vi "Flightsimulator_S2_3.vi"() -> ()   [LabVIEW 2009]
uses:
  <vilib>/Platform/TimedLoop/XDataNode/XDataNode.xnode
  <vilib>/Platform/TimedLoop/XDataNode/loadlvalarms.vi
  <vilib>/Platform/TimedLoop/XDataNode/timing_clust.ctl
  <vilib>/Platform/TimedLoop/XDataNode/nitl_modes.ctl
  <vilib>/Platform/TimedLoop/XDataNode/wakeup.ctl
  <menus>/Universal Library/Das16.llb/FromEng(single).VI
  <vilib>/Platform/TimedLoop/XDataNode/XDNodeRunTimeDep.lvlib
  <vilib>/ptbypt/NI_PtbyPt.lvlib
panel:
  in  "Protocol123":u16(ring) items=["no color- no switch", "color mode", "no color- switch(black at change)"]
  out "colorchange":bool
  out "OK":bool=TRUE
  out "final test 2":dbl(slide)=-0.5605680868838764 scale=-1.0..1.0
  out "final test 1":dbl(slide)=0.24740124740124741 scale=-1.0..1.0
  out "training short":dbl(slide)=0.9652317880794702 scale=-1.0..1.0
  out "training8":dbl(slide)=0.9652317880794702 scale=-1.0..1.0
  out "training7":dbl(slide)=0.8611570247933884 scale=-1.0..1.0
  out "test3":dbl(slide)=-1.0 scale=-1.0..1.0
  out "training6":dbl(slide)=-0.21869782971619364 scale=-1.0..1.0
  out "training5":dbl(slide)=0.8540268456375839 max=5.904801692781309e-210 step=1.08742394e-315 scale=-1.0..1.0
  out "test 2":dbl(slide)=-0.6904962153069807 scale=-1.0..1.0
  out "test 1":dbl(slide)=-0.1886949293433084 scale=-1.0..1.0
  out "training 4":dbl(slide)=1.0 scale=-1.0..1.0
  out "training 3":dbl(slide)=1.0 scale=-1.0..1.0
  out "training 2":dbl(slide)=-0.2332214765100671 scale=-1.0..1.0
  out "training 1":dbl(slide)=0.03096234309623431 scale=-1.0..1.0
  out "pretest 2":dbl(slide)=-0.5708367854183927 scale=-1.0..1.0
  out "pretest 1":dbl(slide)=-0.26220016542597185 scale=-1.0..1.0
  out "protocol":string="nocolor mode"
  out "protocol 2":u16(ring)=1 items=["Switch mode", "color mode", "other"]
  in  "color":bool
  out "color when positive":string="green"
  in  "add to datainput":dbl
  in  "add period":dbl
  in  "forcelaseroffmanual":bool
  in  "minimumtotorquenotflying":ext
  in  "torquenotflying":ext=-6.216083831386964
  in  "beep":bool
  out "datatest":dbl=0.7859212239583333
  in  "DTC":bool=TRUE
  in  "minimum for not flying":ext=0.03
  in  "remarks":string="change in gain?"
  out "sleft01_right0-1":i32=-1
  out "period":i32=-12648 step=206880616
  out "ErrCode 3":i32
  out "laser power real":dbl=2.1
  in  "laser power 0-41":dbl=29.0
  in  "force laser on":bool
  out "laserison":bool
  out "laser":bool
  out "ErrCode 2":i32
  out "ErrCode":i32
  out "PULSE":bool
  out "error out 3":errorcluster
  in  "force end of exp":bool
  out "Elapsed Time (s) 2":dbl(slide)=43.1674690246582 caption="Elapsed Time (s)" max=1.19698869e-315 scale=0.12..120.0
  out "Score 2":dbl=0.17155756207674944
  out "Histogram 2":dynamicdata(graph)=[{"t0"=timestamp(-4.833333333333333 s since 1904-01-01), "dt"=0.3333333333333333, "Y"=[0.0, 0.0, 1.0, 3.0, 5.0, 9.0, 19.0, 14.0, 25.0, 26.0, 42.0, 53.0, 52.0, 68.0, 50.0, 11.0, 12.0, 28.0, 15.0, 30.0, 27.0, 39.0, 57.0, 65.0, 78.0, 157.0, 0.0, 0.0, 0.0, 0.0], "attributes"=variant("NI_ChannelName"=variant(string " (Histogram)"), "NI_ExpIsRelativeTime"=variant(bool TRUE), "NI_ExpStartTimeStamp"=variant(timestamp timestamp(0 s since 1904-01-01)), "NI_ExpTimeStamp"=variant(timestamp timestamp(3352812616.4418974 s since 1904-01-01)), "NI_ExpXDimension"=variant(string "BIN"), "NI_OriginalChannelName"=variant(string ""))}] caption="Histogram"
  out "Waveform Chart 3":ext(graph)=0.7863281249999999889
  out "end of experiment":bool
  out "punished":string="positive-left"
  out "Eng Units":sgl=0.78632814
  in  "serie(s)":dbl=60.0
  in  "genotype":string="wtb"
  in  "Path":path=path "D:/dokumente/data/FSdata/switcheffect/switch.txt"
  in  "side punished":bool=TRUE
  in  "start":bool
  # "left"
  # "right"
  # "x"
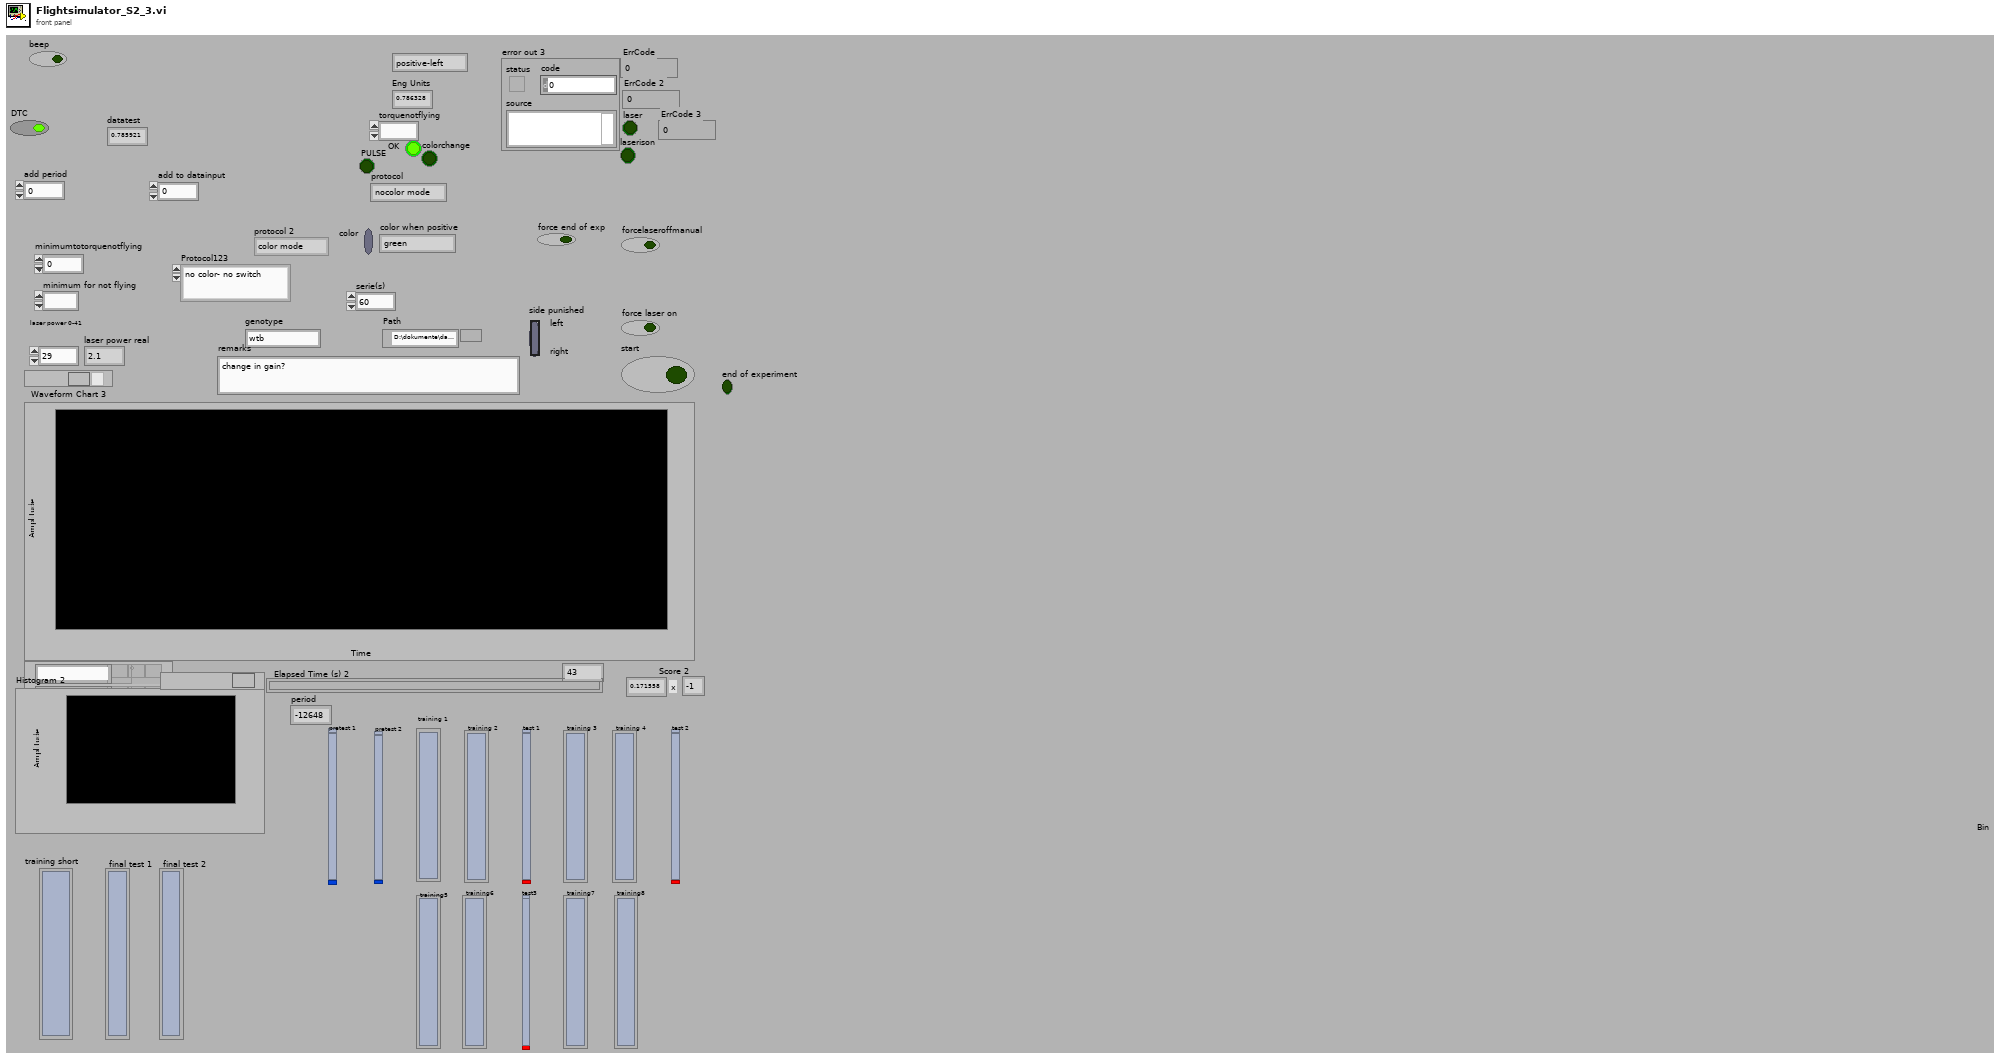
[diagram p1: front panel]
types:
  T1 = typedef "XDNodeRunTimeDep.lvlib/timing_clust.ctl" = cluster{"Expected End [f-1]":u64, "Actual End [f-1]":u64, "Finished Late? [f-1]":bool, "Expected End [i-1]":u64, "Actual End [i-1]":u64, "Finished Late? [i-1]":bool, "Expected Start [i]":u64, "Actual Start [i]":u64, "Expected Start [f]":u64, "Actual Start [f]":u64, "Source Name":string, "Structure Name":string, "Period":i64, "Deadline":i64, "Offset":i64, "Start":i64, "Priority":i32, "Timeout":i32, "Mode":T2, "Wakeup Reason":T3, "Error":errorcluster, "Source Type":string, "Secondary Source Type":string, "Global End Time":u64, "Global Start Time":u64, "Frame Duration":u64, "Iteration Duration":u64, "Assigned CPU":i32, "I/O Scan Engine Mode":u32}
  T2 = typedef "XDNodeRunTimeDep.lvlib/nitl_modes.ctl" = enum32{"No Change", "Process missed periods, maintain original phase", "Discard missed periods, maintain original phase", "Process missed periods, ignore original phase", "Discard missed periods, ignore original phase"}
  T3 = typedef "XDNodeRunTimeDep.lvlib/wakeup.ctl" = enum32{"Normal", "Aborted", "Asynchronous wakeup", "Timing source error", "Timed loop error", "Timeout"}
  T4 = enum16{"open", "replace", "create", "open or create", "replace or create", "replace or create with confirmation"}
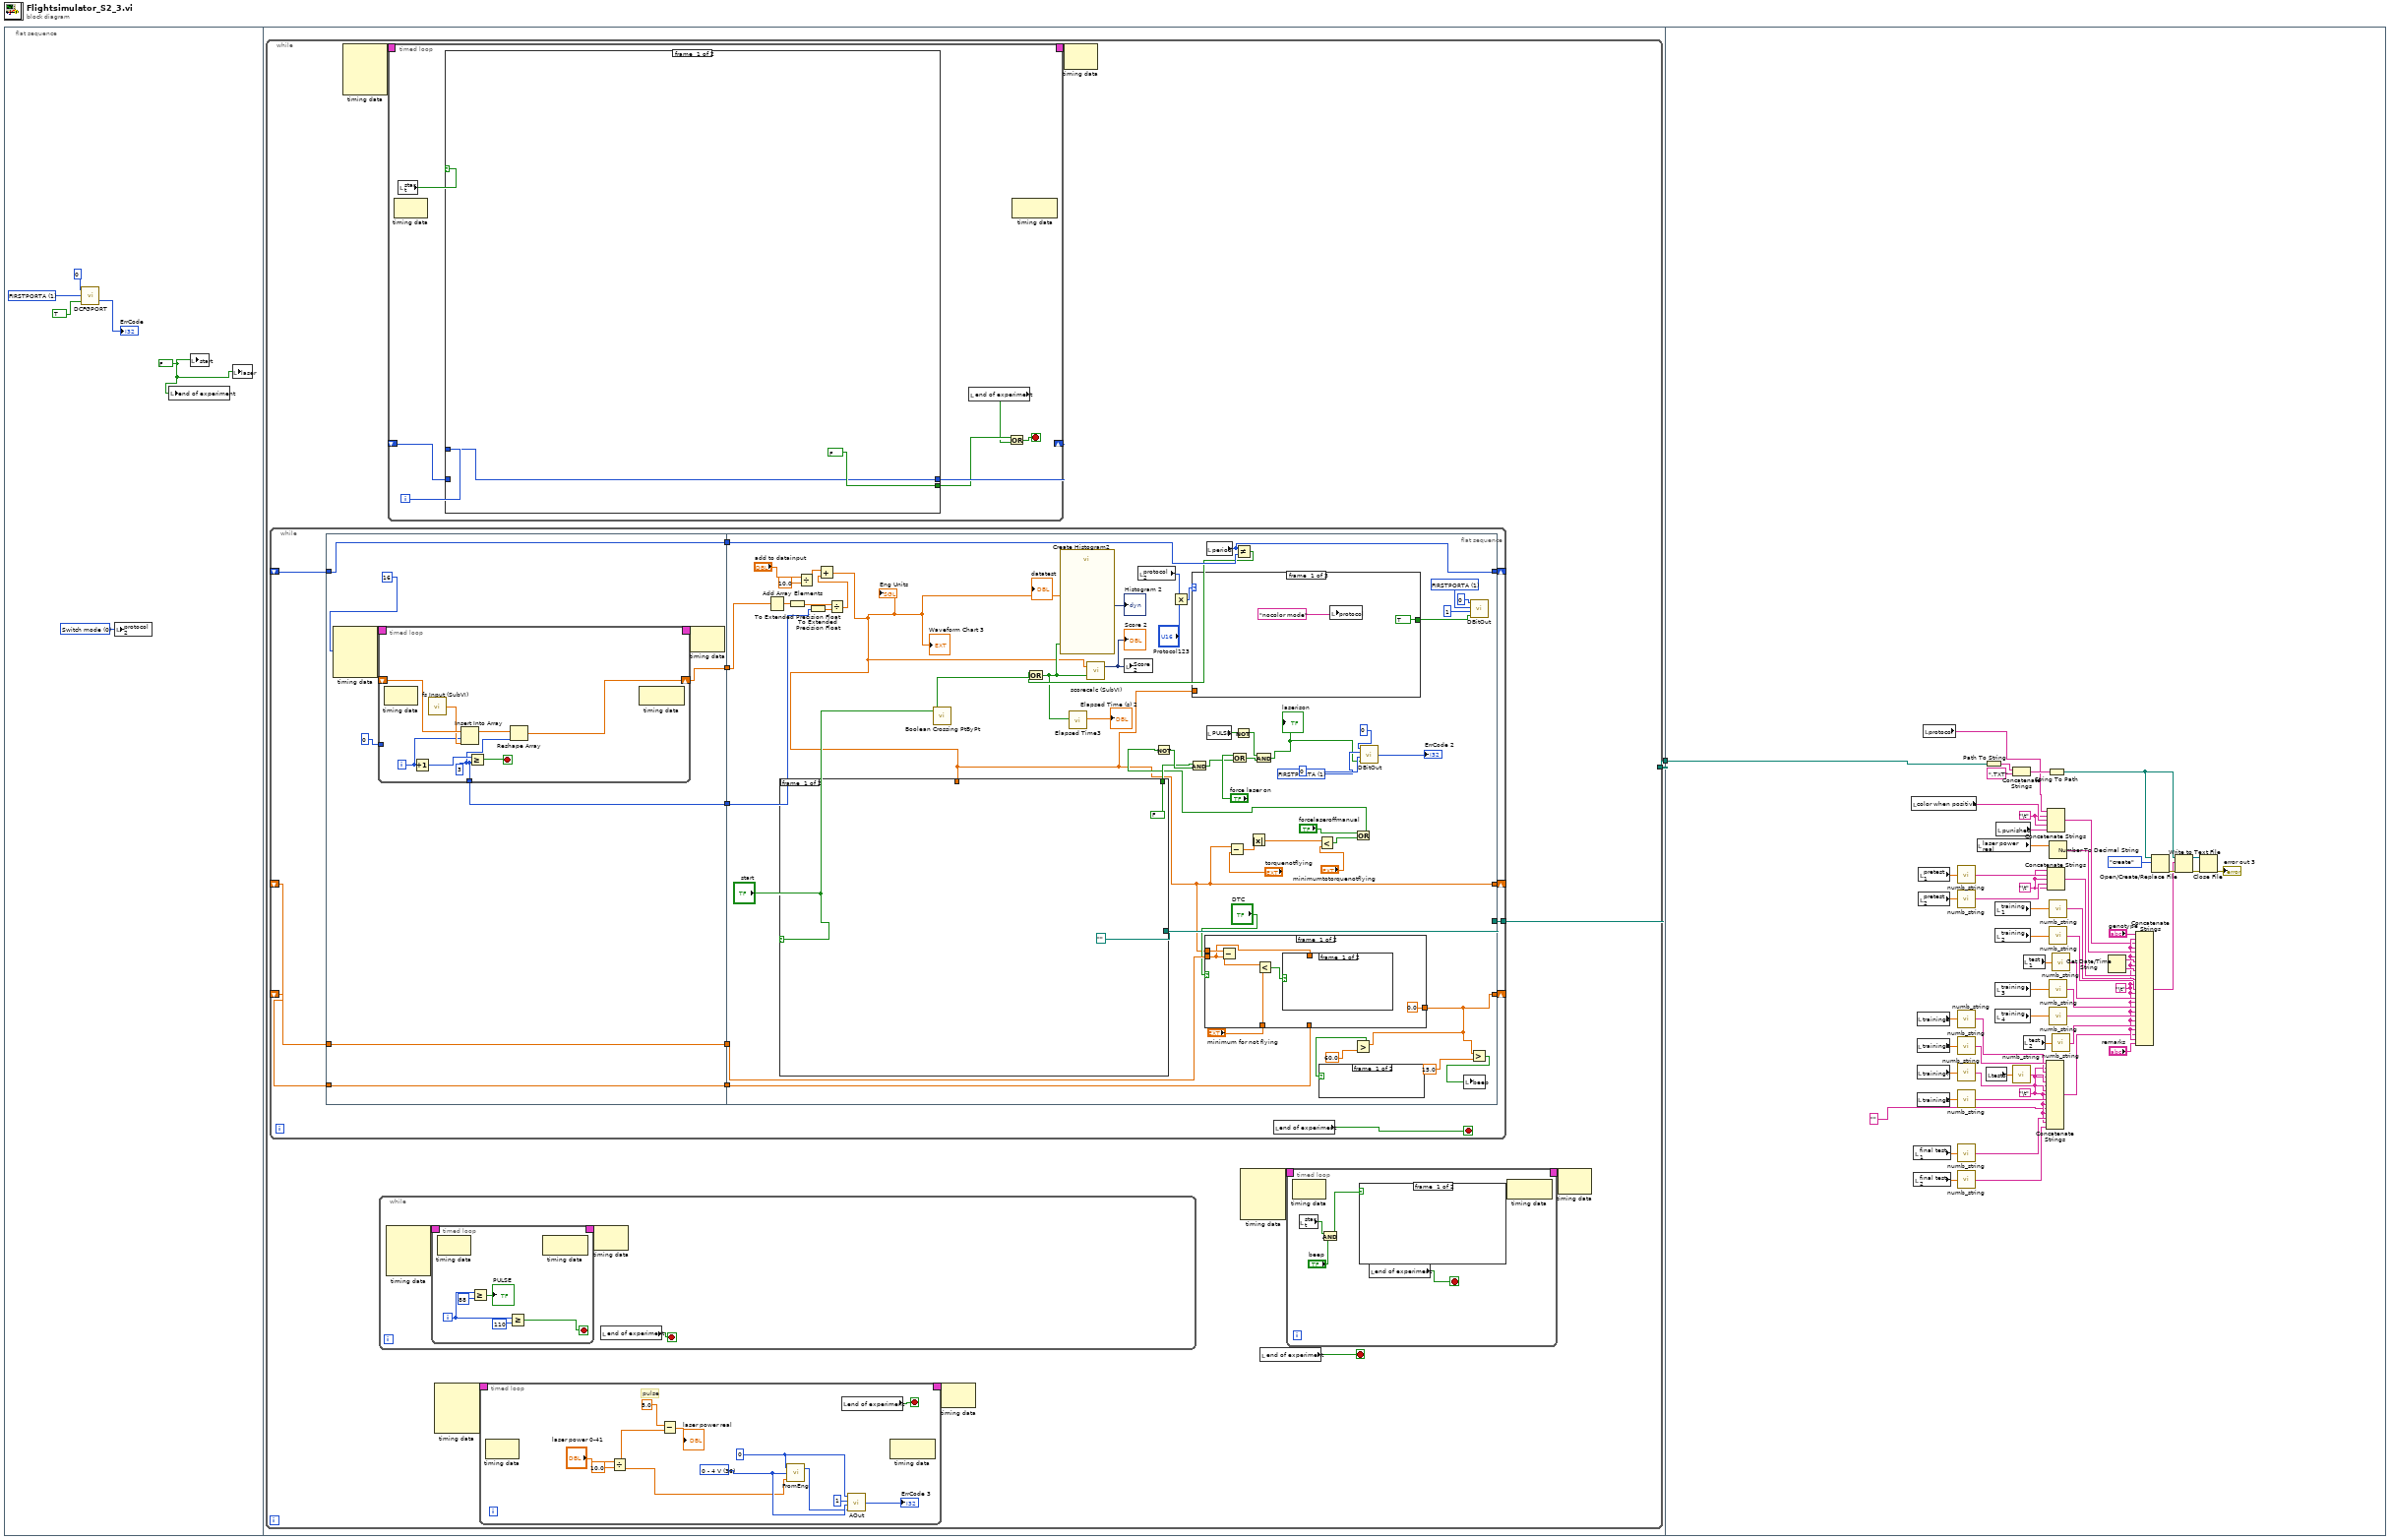
[diagram p0: block diagram]
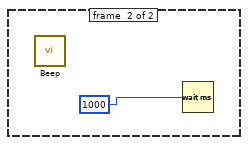
[diagram p2: hidden frame]
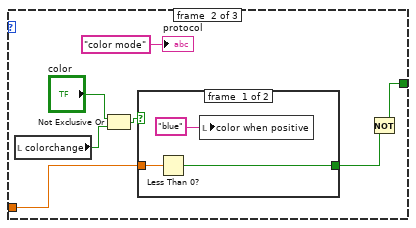
[diagram p3: hidden frame]
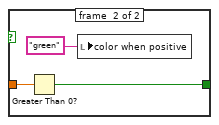
[diagram p4: hidden frame]
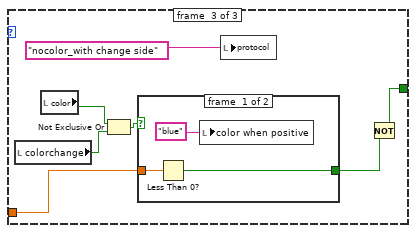
[diagram p5: hidden frame]
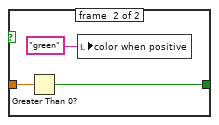
[diagram p6: hidden frame]
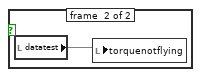
[diagram p7: hidden frame]
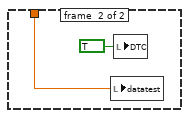
[diagram p8: hidden frame]
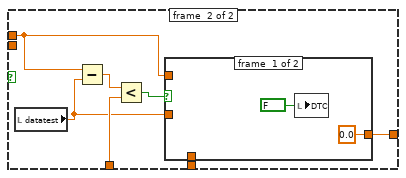
[diagram p9: hidden frame]
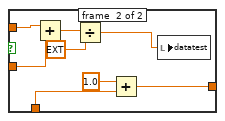
[diagram p10: hidden frame]
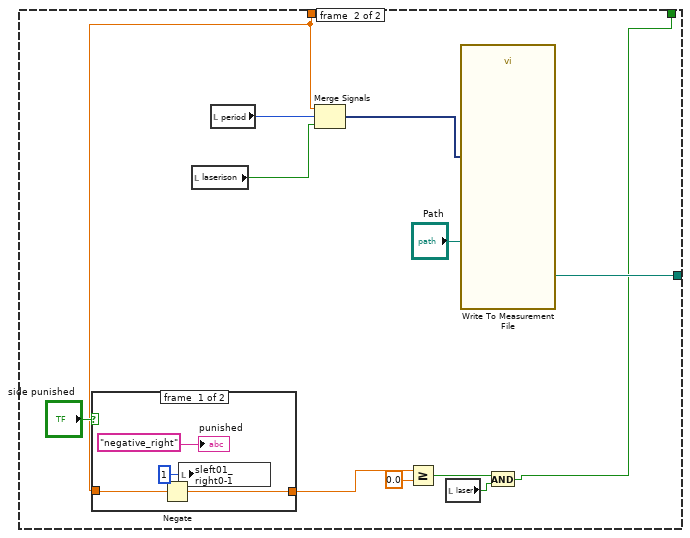
[diagram p11: hidden frame]
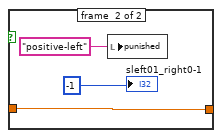
[diagram p12: hidden frame]
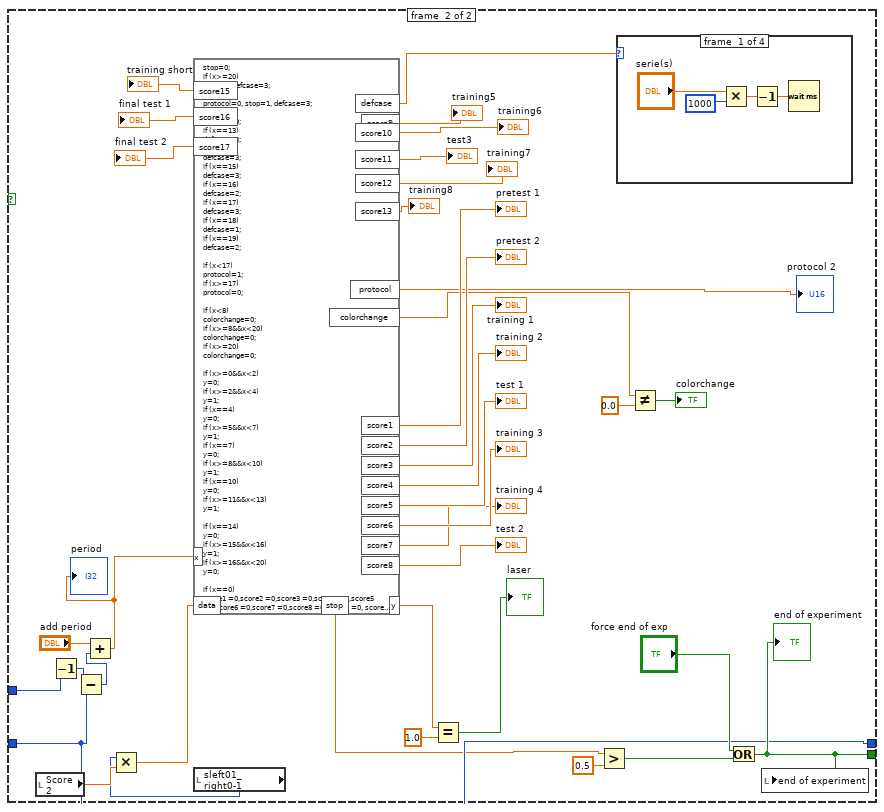
[diagram p13: hidden frame]
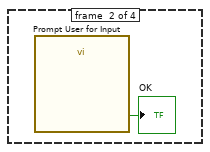
[diagram p14: hidden frame]
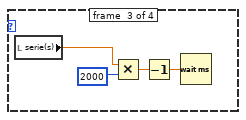
[diagram p15: hidden frame]
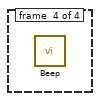
[diagram p16: hidden frame]
diagram:
  n1 = flat-sequence {
    tunnel: [w8] -> w1
    tunnel: w1 -> [w316]
    frame #0 {
      w2 = u16 0 items=["Switch mode", "color mode", "other"] ("protocol 2")
      w6 = 1 items=["AUXPORT", "FIRSTPORTA", "FIRSTPORTB", "FIRSTPORTCL", "FIRSTPORTCH", "SECONDPORTA", "SECONDPORTB", "SECONDPORTCL", "SECONDPORTCH", "THIRDPORTA", "THIRDPORTB", "THIRDPORTCL", "THIRDPORTCH", "FOURTHPORTA", "FOURTHPORTB", "FOURTHPORTCL", "FOURTHPORTCH", "FIFTHPORTA", "FIFTHPORTB", "FIFTHPORTCL", "FIFTHPORTCH", "SIXTHPORTA", "SIXTHPORTB", "SIXTHPORTCL", "SIXTHPORTCH", "SEVENTHPORTA", "SEVENTHPORTB", "SEVENTHPORTCL", "SEVENTHPORTCH", "EIGTHPORTA", "EIGHTHPORTB", "EIGHTHPORTCL", "EIGHTHPORTCH"] ("PortNum")
      w3 = FALSE
      n2 = call <menus>:"DCFGPORT.VI"("Direction"=TRUE, "PortNum"=w6, "BoardNum"=u32 0) -> ("ErrCode"=→"ErrCode":i32)  [unwired: 1 out]
      n3 = local write "protocol 2"(w2) -> ()
      n4 = local write "end of experiment"(w3) -> ()
      n5 = local write "start"(w3) -> ()
      n6 = local write "laser"(w3) -> ()
    }
    frame #1 {
      n7 = while {
        tunnel: [w11] -> w8
        stop <- w14 stop-if-true
        n8 = while {
          tunnel: [w53] -> w11
          shift-right: [w51] -> _
          shift-left: _ -> [w50]
          shift-right: [w46] -> _
          shift-left: _ -> [w44]
          shift-right: [w43] -> _
          shift-left: _ -> [w41]
          stop <- w52 stop-if-true
          n9 = flat-sequence {
            tunnel: [w60] -> w49
            tunnel: [w59] -> w48
            tunnel: [w56] -> w47
            tunnel: w50 -> [w56]
            tunnel: [w55] -> w45
            tunnel: w44 -> [w55]
            tunnel: [w54] -> w42
            tunnel: w41 -> [w54]
            tunnel: [w131] -> w53
            tunnel: w49 -> [w124]
            tunnel: w48 -> [w123]
            tunnel: [w116] -> w51
            tunnel: w47 -> [w115]
            tunnel: [w87] -> w46
            tunnel: w45 -> [w107]
            tunnel: [w98] -> w43
            tunnel: w42 -> [w105]
            frame #0 {
              n10 = node-c288(i64 16 ("Period")) -> (w62:T1)  [unwired: 3 in]
              n11 = timed-loop {
                tunnel: 0 ("y") -> [_]
                shift-right: [w66] -> w60
                shift-left: _ -> [w69]
                timing: w62 -> [_]
                timing-out: [_] -> w61
                tunnel: [w63] -> w59
                i -> [w64]
                stop <- w70 stop-if-true
                w63 = 3 ("y")
                n12 = node-c288() -> ()  [unwired: 1 in, 1 out]
                n13 = Increment(x=w64) -> (x+1=w65:i32)
                n14 = call "fs Input (SubVI).vi"() -> ("Eng Units"=w68:sgl)  [unwired: 1 out]
                n15 = Insert Into Array(array=w69, index=w64, new element=w68) -> (w67:sgl[])
                n16 = Greater Or Equal?(x=w65, y=w63) -> (x >= y?=w70:bool)
                n17 = Reshape Array(w67, w63) -> (w66:sgl[])
                n18 = node-c288() -> ()  [unwired: 1 in, 1 out]
              }
              n19 = node-c288(w61) -> ()  [unwired: 1 out]
            }
            frame #1 {
              w84 = u32 1 items=["AUXPORT", "FIRSTPORTA"] ("PortType")
              w120 = u32 1 items=["AUXPORT", "FIRSTPORTA"] ("PortType")
              n20 = Add Array Elements(numeric array=w124) -> (sum=w127:sgl)
              n21 = To Extended Precision Float(1:w127) -> (0:w125:ext)
              n22 = Divide(x="add to datainput", y=10.0) -> (x/y=w79:dbl)
              n23 = To Extended Precision Float(1:w123) -> (0:w126:ext)
              n24 = Divide(x=w125, y=w126) -> (x/y=w88:ext)
              n25 = Add(x=w79, y=w88) -> (x+y=w87:ext)
              "Eng Units" <- w87
              "Waveform Chart 3" <- w87
              n26 = case shown="True" "start" {
                tunnel: w87 -> [_ w191]
                tunnel: [path "" ("Filename Out") w197] -> w131
                tunnel: [FALSE w188] -> w100
                frame #0 {
                }
                frame #1 {
                  n27 = case shown="False" "side punished" {
                    tunnel: w191 -> [w203 w206]
                    tunnel: [w201 w206] -> w196
                    frame #0 {
                      n28 = Negate(x=w203) -> (-x=w201:ext)
                      n29 = local write "sleft01_right0-1"(1 ("sleft01_right0-1")) -> ()
                      "punished" <- "negative_right"
                    }
                    frame #1 {
                      n30 = local write "punished"("positive-left") -> ()
                      "sleft01_right0-1" <- -1
                    }
                  }
                  n31 = local read "laserison"() -> (w189:bool)
                  n32 = local read "period"() -> (w190:i32)
                  n33 = Merge Signals(w191, w190, w189) -> (w198:dynamicdata)
                  n34 = Greater Or Equal?(x=w196, y=sgl 0.0) -> (x >= y?=w193:bool)
                  n35 = local read "laser"() -> (w192:bool)
                  n36 = call "Write To Measurement File"("Signals"=w198, "Filename"="Path") -> ("Filename Out"=w197:path)  [unwired: 15 in, 2 out]
                  n37 = And(x=w193, y=w192) -> (x .and. y?=w188:bool)
                }
              }
              n38 = call <vilib>:"Boolean Crossing PtByPt.vi"("input"="start") -> ("crossing"=w129:bool)  [unwired: 2 in]
              n39 = local read "protocol 2"() -> (w82:u16)
              n40 = Multiply(x="Protocol123", y=w82) -> (x*y=w81:u16)
              n41 = case shown="2" w81 {
                tunnel: w87 -> [_ w138 w152]
                tunnel: [TRUE w136 w151] -> w83
                frame #0 {
                  n42 = local write "protocol"("nocolor mode") -> ()
                }
                frame #1 {
                  n43 = local read "colorchange"() -> (w134:bool)
                  n44 = Not Exclusive Or(1:w134, 2:"color") -> (0:w135:bool)
                  n45 = case shown="True" w135 {
                    tunnel: [w143 w146] -> w140
                    tunnel: w138 -> [w141 w144]
                    frame #0 {
                      n46 = Less Than 0?(x=w141) -> (x < 0?=w143:bool)
                      n47 = local write "color when positive"("blue") -> ()
                    }
                    frame #1 {
                      n48 = Greater Than 0?(x=w144) -> (x > 0?=w146:bool)
                      n49 = local write "color when positive"("green") -> ()
                    }
                  }
                  n50 = Not(x=w140) -> (.not. x?=w136:bool)
                  "protocol" <- "color mode"
                }
                frame #2 {
                  n51 = local read "colorchange"() -> (w149:bool)
                  n52 = local read "color"() -> (w148:bool)
                  n53 = Not Exclusive Or(1:w149, 2:w148) -> (0:w150:bool)
                  n54 = case shown="True" w150 {
                    tunnel: [w156 w159] -> w153
                    tunnel: w152 -> [w154 w157]
                    frame #0 {
                      n55 = Less Than 0?(x=w154) -> (x < 0?=w156:bool)
                      n56 = local write "color when positive"("blue") -> ()
                    }
                    frame #1 {
                      n57 = Greater Than 0?(x=w157) -> (x > 0?=w159:bool)
                      n58 = local write "color when positive"("green") -> ()
                    }
                  }
                  n59 = local write "protocol"("nocolor_with change side") -> ()
                  n60 = Not(x=w153) -> (.not. x?=w151:bool)
                }
              }
              n61 = case shown="True" "DTC" {
                tunnel: "minimum for not flying" -> [w165 w174]
                tunnel: w107 -> [w161 _]
                tunnel: w87 -> [w164 w169]
                tunnel: w105 -> [_ w171]
                tunnel: [0.0 w170] -> w98
                frame #0 {
                  n62 = Subtract(x=w164, y=w161) -> (x-y=w166:ext)
                  n63 = Less?(x=w166, y=w165) -> (x < y?=w163:bool)
                  n64 = case shown="True" w163 {
                    tunnel: w161 -> [_ w167]
                    frame #0 {
                    }
                    frame #1 {
                      n65 = local write "datatest"(w167) -> ()
                      n66 = local write "DTC"(TRUE ("DTC")) -> ()
                    }
                  }
                }
                frame #1 {
                  n67 = local read "datatest"() -> (w172:dbl)
                  n68 = Subtract(x=w169, y=w172) -> (x-y=w175:ext)
                  n69 = Less?(x=w175, y=w174) -> (x < y?=w173:bool)
                  n70 = case shown="True" w173 {
                    tunnel: w172 -> [_ w185]
                    tunnel: w169 -> [_ w184]
                    tunnel: w171 -> [_ w180]
                    tunnel: [0.0 w178] -> w170
                    frame #0 {
                      n71 = local write "DTC"(FALSE ("DTC")) -> ()
                    }
                    frame #1 {
                      n72 = Add(x=w184, y=w185) -> (x+y=w183:ext)
                      n73 = Divide(x=w183, y=ext 2.0) -> (x/y=w181:ext)
                      n74 = Add(x=1.0, y=w180) -> (x+y=w178:dbl)
                      n75 = local write "datatest"(w181) -> ()
                    }
                  }
                }
              }
              n76 = local read "period"() -> (w116:i32)
              n77 = local read "PULSE"() -> (w114:bool)
              n78 = Subtract(x=w87, y="torquenotflying") -> (x-y=w94:ext)
              n79 = Not(x=w114) -> (.not. x?=w113:bool)
              n80 = Not Equal?(x=w116, y=w115) -> (x != y?=w110:bool)
              n81 = Or(x=w110, y=w129) -> (x .or. y?=w103:bool)
              n82 = call "Create Histogram2"("Reset"=w103, "Signal"=w87) -> ("Histogram"=→"Histogram 2":dynamicdata)  [unwired: 8 in, 1 out]
              n83 = call "Elapsed Time3"("Reset"=w103) -> ("Elapsed Time (s)"=→"Elapsed Time (s) 2":dbl)  [unwired: 11 in, 7 out]
              n84 = call "scorecalc (SubVI).vi"("Reset"=w103, "Slide"=w87) -> ("Dynamic Data"=w128:dynamicdata)  [unwired: 1 out]
              "Score 2" <- w128
              n85 = local write "Score 2"(w128) -> ()
              n86 = Absolute Value(x=w94) -> (abs(x)=w89:ext)
              n87 = Less?(x=w89, y="minimumtotorquenotflying") -> (x < y?=w92:bool)
              n88 = Or(x="forcelaseroffmanual", y=w92) -> (x .or. y?=w90:bool)
              n89 = Not(x=w90) -> (.not. x?=w109:bool)
              n90 = And(x=w100, y=w109) -> (x .and. y?=w99:bool)
              n91 = Or(x="force laser on", y=w99) -> (x .or. y?=w112:bool)
              n92 = And(x=w113, y=w112) -> (x .and. y?=w101:bool)
              "laserison" <- w101
              n93 = Greater?(x=w98, y=60.0) -> (0:w96:bool)
              n94 = case shown="True" w96 {
                frame #0 {
                }
                frame #1 {
                  n95 = local read "datatest"() -> (w160:dbl)
                  n96 = local write "torquenotflying"(w160) -> ()
                }
              }
              n97 = call <menus>:"DBitOut.VI"("BitValue"=w101, "BitNum"=u32 0, "PortType"=w120, "BoardNum"=u32 0) -> ("ErrCode"=→"ErrCode 2":i32)
              n98 = Greater?(x=w98, y=15.0) -> (0:w102:bool)
              n99 = local write "beep"(w102) -> ()
              n100 = call <menus>:"DBitOut.VI"("BitValue"=w83, "BitNum"=u32 1, "PortType"=w84, "BoardNum"=u32 0) -> ()  [unwired: 1 out]
            }
          }
          n101 = local read "end of experiment"() -> (w52:bool)
        }
        n102 = node-c288() -> (w16:T1)  [unwired: 4 in]
        n103 = while {
          stop <- w207 stop-if-true
          n104 = node-c288() -> (w209:T1)  [unwired: 4 in]
          n105 = timed-loop {
            timing: w209 -> [_]
            timing-out: [_] -> w208
            i -> [w212]
            stop <- w210 stop-if-true
            n106 = node-c288() -> ()  [unwired: 1 in, 1 out]
            n107 = Greater Or Equal?(x=w212, y=88 ("SIZE1")) -> (x >= y?=→"PULSE":bool)
            n108 = Greater Or Equal?(x=w212, y=110 ("RESET PULSE")) -> (x >= y?=w210:bool)
            n109 = node-c288() -> ()  [unwired: 1 in, 1 out]
          }
          n110 = node-c288(w208) -> ()  [unwired: 1 out]
          n111 = local read "end of experiment"() -> (w207:bool)
        }
        n112 = timed-loop {
          timing: w16 -> [_]
          timing-out: [_] -> w15
          shift-right: [w222] -> _
          shift-left: _ -> [w223]
          i -> [w224]
          stop <- w220 stop-if-true
          n113 = node-c288() -> ()  [unwired: 1 in, 1 out]
          n114 = local read "start"() -> (w225:bool)
          n115 = case shown="True" w225 {
            tunnel: [FALSE w263] -> w221
            tunnel: w224 -> [w226 w261]
            tunnel: w223 -> [_ w257]
            tunnel: [w226 w257] -> w222
            frame #0 {
            }
            frame #1 {
              n116 = local read "Score 2"() -> (w264:dbl)
              n117 = Decrement(x=w261) -> (x-1=w260:i32)
              n118 = Subtract(x=w260, y=w257) -> (x-y=w253:i32)
              n119 = Add(x="add period", y=w253) -> (x+y=w233:dbl)
              "period" <- w233
              n120 = local read "sleft01_right0-1"() -> (w256:i32)
              n121 = Multiply(x=w256, y=w264) -> (x*y=w234:dbl)
              n122 = formula code="stop=0;\nif (x>=20)\nstop=1, defcase=3;\nif (x<0)\nprotocol=0, stop=1, defcase=3;\nif (x<13)\ndefcase=0;\nif (x==13)\ndefcase=3;\nif (x==14)\ndefcase=3;\nif (x==15)\ndefcase=3;\nif (x==16)\ndefcase=2;\nif (x==17)\ndefcase=3;\nif (x==18)\ndefcase=1;\nif (x==19)\ndefcase=2;\n\nif (x<17)\nprotocol=1;\nif (x>=17)\nprotocol=0;\n\nif (x<8)\ncolorchange=0;\nif (x>=8&&x<20)\ncolorchange=0;\nif (x>=20)\ncolorchange=0;\n\nif (x>=0&&x<2)\ny=0;\nif (x>=2&&x<4)\ny=1;\nif (x==4)\ny=0;\nif (x>=5&&x<7)\ny=1;\nif (x==7)\ny=0;\nif (x>=8&&x<10)\ny=1;\nif (x==10)\ny=0;\nif (x>=11&&x<13)\ny=1;\n\nif (x==14)\ny=0;\nif (x>=15&&x<16)\ny=1;\nif (x>=16&&x<20)\ny=0;\n\nif (x==0)\nscore1 =0,score2 =0,score3 =0,score4 =0,score5 =0,score6 =0,score7 =0,score8 =0,score9 =0, score10 =0,\nscore11 =0,score12 =0,score13 =0,score15 =0,score16 =0,score17 =0;\nif (x==1)\nscore1 = data;\nif (x==2)\nscore2 = data;\nif (x==3)\nscore3 = data;\nif (x==4)\nscore4 = data;\nif (x==5)\nscore5 = data;\nif (x==6)\nscore6 = data;\nif (x==7)\nscore7 = data;\nif (x==8)\nscore8 = data;\n\nif (x==9)\nscore9 = data;\nif (x==10)\nscore10 = data;\nif (x==11)\nscore11 = data;\nif (x==12)\nscore12 = data;\nif (x==13)\nscore13 = data;\n\n\nif (x==16)\nscore15 = data;\nif (x==17)\nscore16 = data;\nif (x==20)\nscore17 = data;"("x"=w233, "data"=w234) -> ("score2"=→"pretest 2":dbl, "stop"=w235:dbl, "score1"=→"pretest 1":dbl, "score3"=→"training 1":dbl, "score4"=→"training 2":dbl, "score5"=→"test 1":dbl, "score6"=→"training 3":dbl, "score7"=→"training 4":dbl, "score8"=→"test 2":dbl, "score9"=→"training5":dbl, "y"=w236:dbl, "defcase"=w232:dbl, "score10"=→"training6":dbl, "score11"=→"test3":dbl, "score12"=→"training7":dbl, "score13"=→"training8":dbl, "score16"=→"final test 1":dbl, "score17"=→"final test 2":dbl, "score15"=→"training short":dbl, "protocol"=→"protocol 2":dbl, "colorchange"=w231:dbl)
              n123 = Equal?(x=w236, y=1.0) -> (x = y?=→"laser":bool)
              n124 = Greater?(x=w235, y=0.5) -> (0:w255:bool)
              n125 = case shown="3.." w232 {
                frame #0 {
                  n126 = Multiply(x="serie(s)", y=1000 ("Numeric 2")) -> (x*y=w268:dbl)
                  n127 = Decrement(x=w268) -> (x-1=w267:dbl)
                  n128 = Wait (ms)(milliseconds to wait=w267) -> ()  [unwired: 1 out]
                }
                frame #1 {
                  n129 = call "Prompt User for Input"() -> ("OK"=→"OK":bool)  [unwired: 18 in, 1 out]
                }
                frame #2 {
                  n130 = local read "serie(s)"() -> (w271:dbl)
                  n131 = Multiply(x=w271, y=2000 ("Numeric 2")) -> (x*y=w273:dbl)
                  n132 = Decrement(x=w273) -> (x-1=w272:dbl)
                  n133 = Wait (ms)(milliseconds to wait=w272) -> ()  [unwired: 1 out]
                }
                frame #3 {
                  n134 = call <vilib>:"Beep.vi"() -> ()  [unwired: 12 in]
                }
              }
              n135 = Not Equal?(x=w231, y=0.0) -> (x != y?=→"colorchange":bool)
              n136 = Or(x="force end of exp", y=w255) -> (x .or. y?=w263:bool)
              "end of experiment" <- w263
              n137 = local write "end of experiment"(w263) -> ()
            }
          }
          n138 = local read "end of experiment"() -> (w219:bool)
          n139 = Or(x=w221, y=w219) -> (x .or. y?=w220:bool)
          n140 = node-c288() -> ()  [unwired: 1 in, 1 out]
        }
        n141 = node-c288() -> (w13:T1)  [unwired: 4 in]
        n142 = timed-loop {
          timing: w13 -> [_]
          timing-out: [_] -> w12
          stop <- w36 stop-if-true
          w26 = u32 0 ("BoardNum")
          w34 = 36 items=["Not Programmable"=0, "+- 20 V"=27, "+- 10 V"=1, "+- 5 V"=2, "+- 4 V"=28, "+- 2.5 V"=3, "+- 2 V"=29, "+- 1.67 V"=4, "+- 1.25 V"=5, "+- 1 V"=6, "+- .625 V"=7, "+- .5 V"=8, "+- .25 V"=30, "+- .2 V"=31, "+- .1 V"=9, "+- .05 V"=10, "+- .01 V"=11, "+- .005 V"=12, "0 - 10 V"=13, "0 - 5 V"=14, "0 - 4 V"=36, "0 - 2.5 V"=15, "0 - 2 V"=16, "0 - 1.67 V"=17, "0 - 1.25 V"=18, "0 - 1 V"=19, "0 - .5 V"=32, "0 - .25 V"=33, "0 - .2 V"=34, "0 - .1 V"=20, "0 - .02 V"=35, "0 - .01 V"=21, "4 - 20 mA"=22, "2 - 10 mA"=23, "1 - 5 mA"=24, ".5 - 2.5 mA"=25, "0 - 20 mA"=26] ("Range")
          # "pulse"
          n143 = node-c288() -> ()  [unwired: 1 in, 1 out]
          n144 = Divide(x="laser power 0-41", y=10.0) -> (x/y=w33:dbl)
          n145 = Subtract(x=5.0, y=w33) -> (x-y=→"laser power real":dbl)
          n146 = call-poly <menus>:"FromEng.VI"("Eng Units"=w33, "Range"=w34, "BoardNum (0)"=w26) -> ("DA Data"=w32:u16)  [unwired: 1 out]
          n147 = local read "end of experiment"() -> (w36:bool)
          n148 = call <menus>:"AOut.VI"("DataValue"=w32, "Range"=w34, "Channel"=1, "BoardNum"=w26) -> ("ErrCode"=→"ErrCode 3":i32)
          n149 = node-c288() -> ()  [unwired: 1 in, 1 out]
        }
        n150 = node-c288(w12) -> ()  [unwired: 1 out]
        n151 = node-c288(w15) -> ()  [unwired: 1 out]
        n152 = node-c288() -> (w10:T1)  [unwired: 4 in]
        n153 = local read "end of experiment"() -> (w14:bool)
        n154 = timed-loop {
          timing: w10 -> [_]
          timing-out: [_] -> w9
          stop <- w20 stop-if-true
          n155 = node-c288() -> ()  [unwired: 1 in, 1 out]
          n156 = local read "start"() -> (w17:bool)
          n157 = And(x=w17, y="beep") -> (x .and. y?=w18:bool)
          n158 = case shown="True" w18 {
            frame #0 {
            }
            frame #1 {
              n159 = call <vilib>:"Beep.vi"() -> ()  [unwired: 12 in]
              n160 = Wait (ms)(milliseconds to wait=1000 ("Numeric 2")) -> ()  [unwired: 1 out]
            }
          }
          n161 = local read "end of experiment"() -> (w20:bool)
          n162 = node-c288() -> ()  [unwired: 1 in, 1 out]
        }
        n163 = node-c288(w9) -> ()  [unwired: 1 out]
      }
    }
    frame #2 {
      w282 = "\t"
      w307 = "\t"
      w312 = "\t"
      w310 = "\t"
      n164 = local read "color when positive"() -> (w308:string)
      n165 = local read "final test 1"() -> (w293:dbl)
      n166 = local read "final test 2"() -> (w294:dbl)
      n167 = local read "training5"() -> (w291:dbl)
      n168 = local read "training6"() -> (w292:dbl)
      n169 = local read "training7"() -> (w296:dbl)
      n170 = local read "training8"() -> (w295:dbl)
      n171 = local read "pretest 1"() -> (w299:dbl)
      n172 = local read "pretest 2"() -> (w298:dbl)
      n173 = local read "protocol"() -> (w280:string)
      n174 = call "numb_string.vi"("training 1"=w299) -> ("String"=w314:string)
      n175 = call "numb_string.vi"("training 1"=w298) -> ("String"=w313:string)
      n176 = call "numb_string.vi"("training 1"=w291) -> ("String"=w289:string)
      n177 = call "numb_string.vi"("training 1"=w292) -> ("String"=w288:string)
      n178 = call "numb_string.vi"("training 1"=w296) -> ("String"=w286:string)
      n179 = call "numb_string.vi"("training 1"=w295) -> ("String"=w285:string)
      n180 = call "numb_string.vi"("training 1"=w293) -> ("String"=w284:string)
      n181 = call "numb_string.vi"("training 1"=w294) -> ("String"=w283:string)
      n182 = local read "laser power real"() -> (w318:dbl)
      n183 = Path To String(path=w316) -> (string=w334:string)
      n184 = local read "test3"() -> (w290:dbl)
      n185 = local read "training 1"() -> (w304:dbl)
      n186 = local read "training 2"() -> (w303:dbl)
      n187 = local read "training 3"() -> (w301:dbl)
      n188 = local read "training 4"() -> (w300:dbl)
      n189 = local read "punished"() -> (w306:string)
      n190 = Concatenate Strings(w334, ".TXT" ("string")) -> (w336:string)
      n191 = call "numb_string.vi"("training 1"=w290) -> ("String"=w287:string)
      n192 = local read "test 1"() -> (w302:dbl)
      n193 = local read "test 2"() -> (w297:dbl)
      n194 = Concatenate Strings(w289, w282, w288, w282, w287, w282, w286, w282, w285, w282, "" ("String"), w282, w284, w282, w283) -> (w281:string)
      n195 = Concatenate Strings(w280, w307, w308, w307, w306) -> (w305:string)
      n196 = Concatenate Strings(w312, w314, w312, w313, w312) -> (w311:string)
      n197 = String To Path(string=w336) -> (path=w330:path)
      n198 = Number To Decimal String(number=w318) -> (decimal integer string=w317:string)  [unwired: 1 in]
      n199 = call "numb_string.vi"("training 1"=w304) -> ("String"=w324:string)
      n200 = call "numb_string.vi"("training 1"=w303) -> ("String"=w323:string)
      n201 = call "numb_string.vi"("training 1"=w301) -> ("String"=w321:string)
      n202 = call "numb_string.vi"("training 1"=w300) -> ("String"=w320:string)
      n203 = call "numb_string.vi"("training 1"=w302) -> ("String"=w322:string)
      n204 = call "numb_string.vi"("training 1"=w297) -> ("String"=w319:string)
      n205 = Get Date/Time String() -> (date string=w327:string, time string=w325:string)  [unwired: 3 in]
      n206 = Concatenate Strings("genotype", w310, w305, w310, w317, w310, w327, w310, w325, w311, w324, w310, w323, w310, w322, w310, w321, w310, w320, w310, w319, w310, w281, w310, "remarks") -> (w326:string)
      n207 = Open/Create/Replace File(file path (use dialog)=w330, operation (0:open)=T4."create") -> (error out=w331:errorcluster)  [unwired: 4 in, 2 out]
      n208 = Write to Text File(file (use dialog)=w330, text=w326, error in=w331) -> (refnum out=w333:refnum<file>, error out=w332:errorcluster)  [unwired: 1 in, 1 out]
      n209 = Close File(refnum=w333, error in=w332) -> (error out=→"error out 3":errorcluster)  [unwired: 1 out]
    }
  }
